vi "3C Helper - Wrap around.vi"(9 "Range allowed":dbl=10.0, 10 "Min allowed":dbl, 11 "Position in":dbl) -> (3 "Wrapped Position out":dbl)   [LabVIEW 2011]
doc: "Takes an input and moves it into a given range, defined by a minimum and a range size. Designed for inputs that are not very far outside the range."
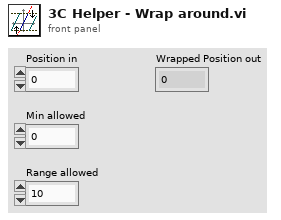
[diagram p1: front panel]
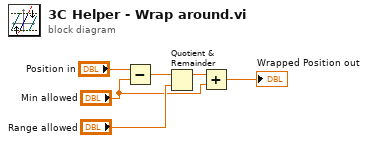
[diagram p0: block diagram]
diagram:
  n1 = Subtract(x="Position in", y="Min allowed") -> (x-y=w5:dbl)
  n2 = Quotient & Remainder(x=w5, y="Range allowed") -> (x-y*floor(x/y)=w3:dbl)  [unwired: 1 out]
  n3 = Add(x=w3, y="Min allowed") -> (x+y=→"Wrapped Position out":dbl)
